vi "Process.vi"(8 "error in (no error)":errorcluster, 10 "Pound in":refnum<class "Pound.lvclass">, 11 "Qbus in":refnum<class "Qbus.lvclass">) -> (0 "error out":errorcluster)   [LabVIEW 2017, in "EmsaAudio.lvlib"]
uses:
  <vilib>/addons/InsightCM/Devices/Shared/Emsa/EmsaAudio/EmsaAudio.lvlib
  <vilib>/addons/Qbus/Qbus.lvclass
  <vilib>/NI/Software Watchdog/Pound/Pound.lvclass
  <vilib>/addons/InsightCM/Devices/Shared/Emsa/EmsaAudio/controls/config.ctl
  <vilib>/addons/TraceLogger/TraceLogger.lvlib
  <vilib>/NI/Software Watchdog/Watchdog/Watchdog.lvclass
  <vilib>/addons/InsightCM/Devices/Shared/Emsa/EmsaAcquisition/EmsaAcquisition.lvlib
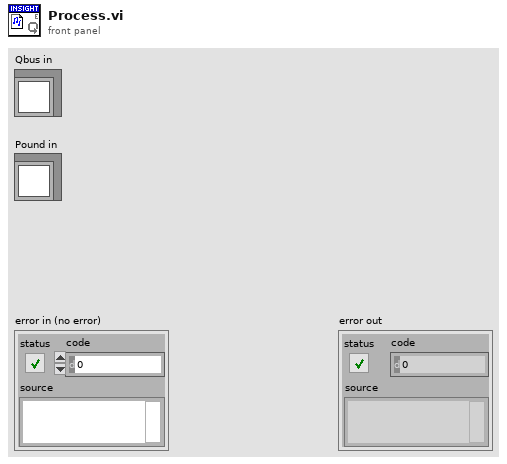
[diagram p1: front panel]
types:
  T1 = typedef "EmsaAudio.lvlib/config.ctl" = cluster{"Active":bool, "Waveform":waveform(dbl), "directory":path, "filenames":string[]}
  T2 = typedef "EmsaAcquisition.lvlib/OnDemandWaveformData.ctl" = cluster{"Channel":string, "First Block":bool, "Last Block":bool, "Center Frequency":dbl, "Waveform":waveform(dbl)}
  T3 = typedef "EmsaAudio.lvlib/AudioFileCompleteBroadcast.ctl" = cluster{"Channel":string, "WAV file path":path}
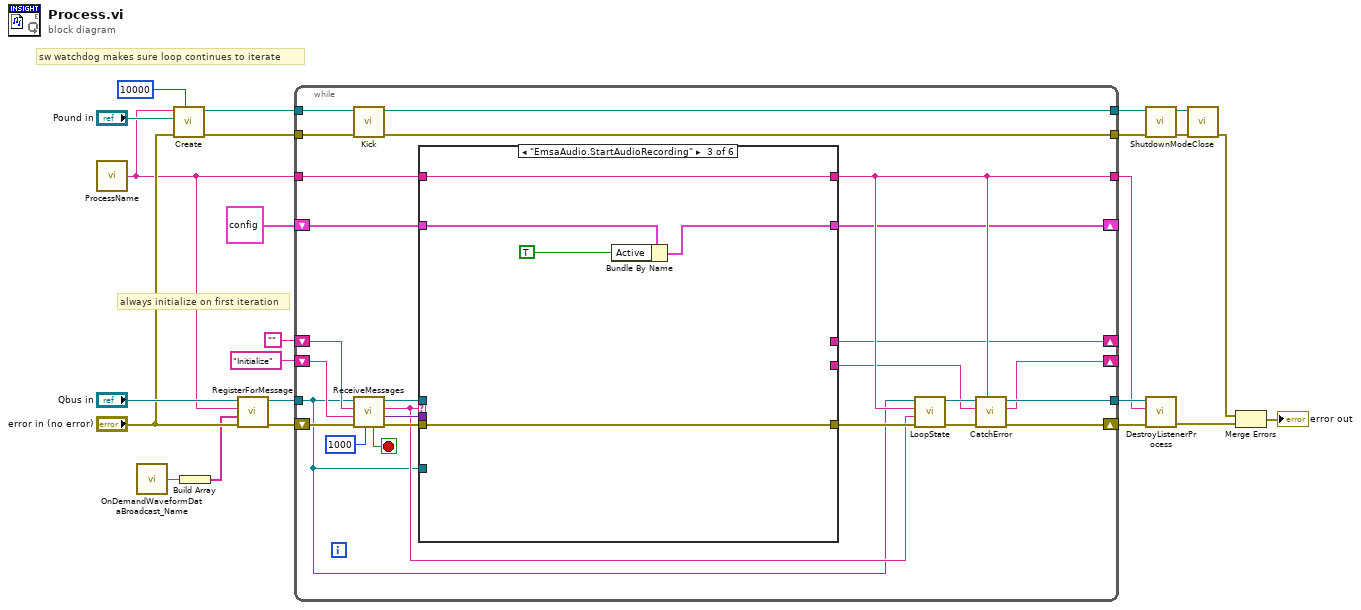
[diagram p0: block diagram]
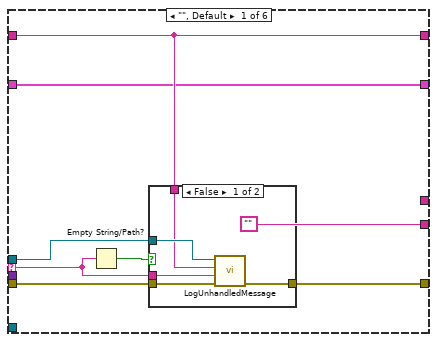
[diagram p2: hidden frame]
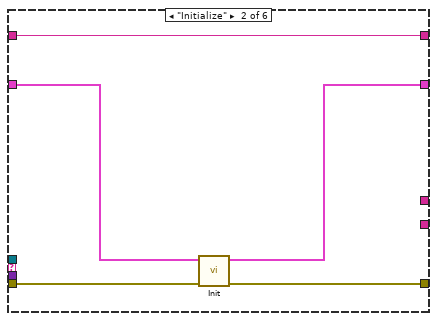
[diagram p4: hidden frame]
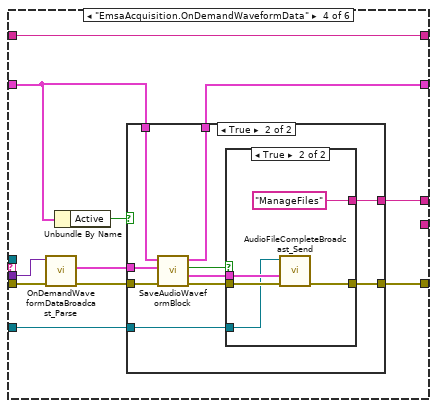
[diagram p5: hidden frame]
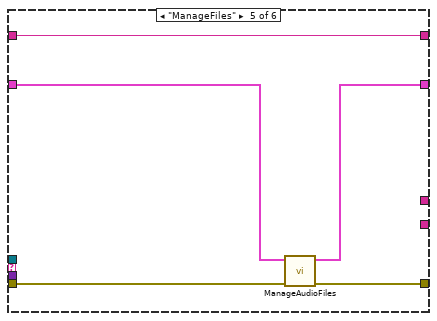
[diagram p8: hidden frame]
diagram:
  # "always initialize on first iteration"
  # "sw watchdog makes sure loop continues to iterate"
  n1 = call <vilib>:"ProcessName.vi"() -> ("process name"=w3:string)  [unwired: 5 in]
  n2 = call <vilib>:"OnDemandWaveformDataBroadcast_Name.vi"() -> ("message name"=w2:string)  [unwired: 5 in]
  n3 = call <vilib>:"Create.vi"("Execution Timeout (ms)"=u32 10000, "error in (no error)"="error in (no error)", "Pound"="Pound in", "Name"=w3) -> ("error out"=w13:errorcluster, "Watchdog"=w19:refnum<data-value>)  [unwired: 6 in]
  n4 = Build Array(w2) -> (w1:string[])
  n5 = call <vilib>:"RegisterForMessage.vi"("error in (no error)"="error in (no error)", "message names"=w1, "process name"=w3, "Qbus in"="Qbus in") -> ("error in (no error)"=w4:errorcluster, "Qbus out"=w6:refnum<class "Qbus.lvclass">)  [unwired: 6 in]
  n6 = while {
    shift-right: [w28] -> _
    shift-left: "" -> [w49]
    tunnel: w6 -> [w25]
    tunnel: w3 -> [w31]
    tunnel: [w43] -> w22
    tunnel: [w30] -> w21
    shift-right: [w42] -> _
    shift-left: "Initialize" -> [w45]
    tunnel: w19 -> [w40]
    tunnel: [w39] -> w15
    tunnel: w13 -> [w38]
    tunnel: [w36] -> w12
    shift-right: [w44] -> w23
    shift-left: w4 -> [w37]
    shift-right: [w26] -> _
    shift-left: T1 {"Active"=FALSE, "Waveform"={"t0"=timestamp(0 s since 1904-01-01), "dt"=1.0, "Y"=[]}, "directory"=path "", "filenames"=[]} ("config") -> [w27]
    stop <- w50 stop-if-true
    n7 = call <vilib>:"Kick.vi"("error in (no error)"=w38, "Watchdog"=w40) -> ("error out"=w36:errorcluster, "Watchdog"=w39:refnum<data-value>)  [unwired: 8 in]
    n8 = call <vilib>:"ReceiveMessages.vi"("Timeout(1000)"=1000 ("milliseconds to wait"), "error in (no error)"=w37, "priority action"=w45, "default action"=w49, "Qbus in"=w25) -> ("error out"=w48:errorcluster, "message value"=w46:variant, "action"=w35:string, "Qbus out"=w47:refnum<class "Qbus.lvclass">, "exit"=w50:bool)  [unwired: 2 in]
    n9 = case shown="\"EmsaAudio.StartAudioRecording\"" w35 {
      selector: w35 -> [w54 _ _ _ _ _]
      tunnel: w48 -> [w57 w68 w70 w82 w107 w111]
      tunnel: w47 -> [w53 _ _ _ _ _]
      tunnel: [w56 w65 w70 w78 w105 w111] -> w41
      tunnel: w46 -> [_ _ _ w83 _ _]
      tunnel: [w52 w69 w74 w85 w108 w110] -> w30
      tunnel: w31 -> [w52 w69 w74 w85 w108 w110]
      tunnel: ["" _ _ _ _ _] -> w29
      tunnel: [_ _ _ w79 _ _] -> w28
      tunnel: w27 -> [w51 w67 w73 w76 w106 w109]
      tunnel: [w51 w66 w72 w84 w104 w109] -> w26
      tunnel: w25 -> [_ _ _ w77 _ _]
      frame "", Default {
        n10 = Empty String/Path?(string/path=w54) -> (empty?=w55:bool)
        n11 = case shown="False" w55 {
          tunnel: [w62 w64] -> w56
          tunnel: w57 -> [w63 w64]
          tunnel: w54 -> [w60 _]
          tunnel: w53 -> [w61 _]
          tunnel: w52 -> [w59 _]
          frame False {
            n12 = call <vilib>:"LogUnhandledMessage.vi"("error in (no error)"=w63, "message"=w60, "process"=w59, "Qbus in"=w61) -> ("error out"=w62:errorcluster)  [unwired: 7 in]
          }
          frame True {
          }
        }
      }
      frame "Initialize" {
        n13 = call <vilib>:"Init.vi"("error in (no error)"=w68, "config in"=w67) -> ("error out"=w65:errorcluster, "config out"=w66:T1)  [unwired: 8 in]
      }
      frame "EmsaAudio.StartAudioRecording" {
        n14 = Bundle By Name(cluster=w73, "Active"=TRUE) -> (w72:T1)
      }
      frame "EmsaAcquisition.OnDemandWaveformData" {
        n15 = call <vilib>:"OnDemandWaveformDataBroadcast_Parse.vi"("error in (no error)"=w82, "message"=w83) -> ("error out"=w81:errorcluster, "on demand waveform"=w80:T2)  [unwired: 8 in]
        n16 = Unbundle By Name(w76) -> ("Active"=w75:bool)
        n17 = case shown="True" w75 {
          tunnel: w76 -> [w87 w97]
          tunnel: [w87 w96] -> w84
          tunnel: w81 -> [w86 w95]
          tunnel: w80 -> [_ w94]
          tunnel: [_ w91] -> w79
          tunnel: [w86 w90] -> w78
          tunnel: w77 -> [_ w88]
          frame False {
          }
          frame True {
            n18 = call <vilib>:"SaveAudioWaveformBlock.vi"("error in (no error)"=w95, "on demand waveform"=w94, "config"=w97) -> ("error out"=w89:errorcluster, "audio file complete"=w92:T3, "complete"=w93:bool, "config"=w96:T1)  [unwired: 5 in]
            n19 = case shown="True" w93 {
              tunnel: w92 -> [_ w100]
              tunnel: [_ "ManageFiles"] -> w91
              tunnel: [w98 w101] -> w90
              tunnel: w89 -> [w98 w102]
              tunnel: w88 -> [_ w99]
              frame False {
              }
              frame True {
                n20 = call <vilib>:"AudioFileCompleteBroadcast_Send.vi"("error in (no error)"=w102, "Audio File Complete"=w100, "Qbus"=w99) -> ("error out"=w101:errorcluster)  [unwired: 7 in, 1 out]
              }
            }
          }
        }
      }
      frame "ManageFiles" {
        n21 = call <vilib>:"ManageAudioFiles.vi"("error in (no error)"=w107, "config"=w106) -> ("error out"=w105:errorcluster, "config out"=w104:T1)  [unwired: 8 in]
      }
      frame "Exit" {
      }
    }
    n22 = call <vilib>:"LoopState.vi"("error in (no error)"=w41, "loop action"=w35, "process name"=w30, "Qbus in"=w25) -> ("error out"=w33:errorcluster, "Qbus out"=w32:refnum<class "Qbus.lvclass">)  [unwired: 6 in]
    n23 = call <vilib>:"CatchError.vi"("source"=w30, "error in (no error)"=w33, "next action in"=w29, "Qbus in"=w32) -> ("error out"=w44:errorcluster, "next action out"=w42:string, "Qbus out"=w43:refnum<class "Qbus.lvclass">)  [unwired: 5 in]
  }
  n24 = call <vilib>:"ShutdownMode.vi"("error in (no error)"=w12, "Watchdog"=w15) -> ("error out"=w14:errorcluster, "Watchdog"=w16:refnum<data-value>)  [unwired: 8 in]
  n25 = call <vilib>:"DestroyListenerProcess.vi"("error in (no error)"=w23, "process name"=w21, "Qbus in"=w22) -> ("error in (no error)"=w11:errorcluster)  [unwired: 7 in, 1 out]
  n26 = call <vilib>:"Close.vi"("error in (no error)"=w14, "Watchdog"=w16) -> ("error out"=w10:errorcluster)  [unwired: 9 in]
  n27 = Merge Errors(w10, w11) -> (→"error out":errorcluster)
